vi "ShooterAxisScaler.vi"(9 "MinValue":dbl, 10 "MaxValue":dbl, 11 "ThrottleAxisIn":dbl) -> (3 "ScaledThrottleOut":dbl)   [LabVIEW 2012]
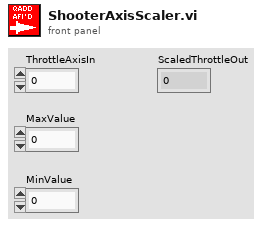
[diagram p1: front panel]
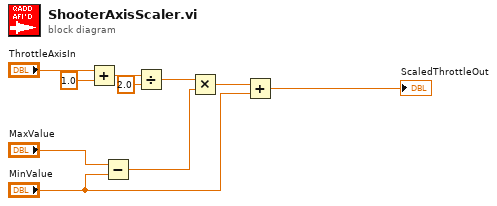
[diagram p0: block diagram]
diagram:
  n1 = Add(x="ThrottleAxisIn", y=1.0) -> (x+y=w8:dbl)
  n2 = Subtract(x="MaxValue", y="MinValue") -> (x-y=w4:dbl)
  n3 = Divide(x=w8, y=2.0) -> (x/y=w5:dbl)
  n4 = Multiply(x=w5, y=w4) -> (x*y=w3:dbl)
  n5 = Add(x=w3, y="MinValue") -> (x+y=→"ScaledThrottleOut":dbl)
